vi "getLevels.vi"(8 "error in (no error)":errorcluster, 11 "DigitalChannel.lvclass in":refnum<class "DigitalChannel.lvclass">) -> (0 "error out":errorcluster, 2 "levels":cluster{"high":dbl, "low":dbl}, 3 "DigitalChannel.lvclass out":refnum<class "DigitalChannel.lvclass">)   [LabVIEW 2009, in "Tools.lvlib" / "DatabaseHelpers.lvlib" / "DigitalChannel.lvclass"]
uses:
  DigitalChannel.lvclass
  DigitalChannel.lvclass/DigitalChannel.ctl
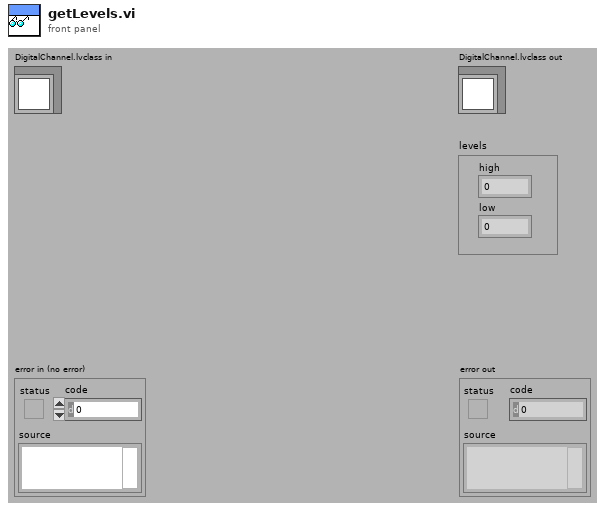
[diagram p1: front panel]
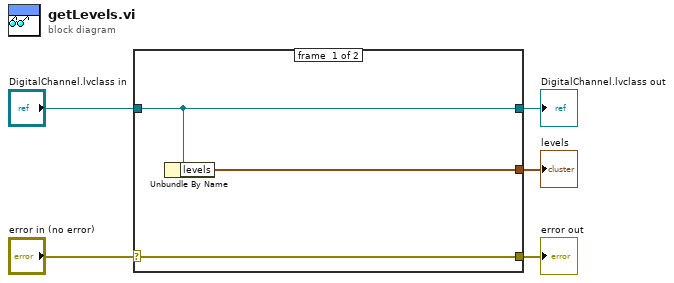
[diagram p0: block diagram]
diagram:
  n1 = case shown="No Error" "error in (no error)" {
    selector: "error in (no error)" -> [w8 w9]
    tunnel: [w8 w9] -> w4
    tunnel: [w7 w10] -> w2
    tunnel: "DigitalChannel.lvclass in" -> [w7 w10]
    tunnel: [w6 _] -> w1
    frame #0 {
      n2 = Unbundle By Name(w7) -> ("levels"=w6:cluster{"high":dbl, "low":dbl})
    }
    frame #1 {
    }
  }
  "error out" <- w4
  "DigitalChannel.lvclass out" <- w2
  "levels" <- w1
